vi "Prioritize LVCAM Error.vi"(10 "Error from LVCAM":errorcluster, 11 "Self Actor in":refnum<class "Self Actor.lvclass">) -> (3 "Self Actor out":refnum<class "Self Actor.lvclass">)   [LabVIEW 2021, in "LVCAM.lvlib" / "Self Actor.lvclass"]
uses:
  Self Actor.lvclass
  Self Actor.lvclass/Self Actor.ctl
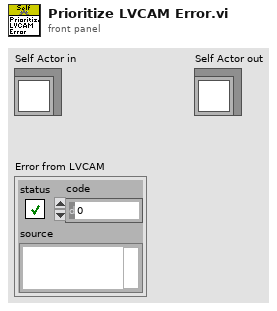
[diagram p1: front panel]
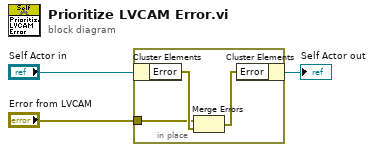
[diagram p0: block diagram]
diagram:
  n1 = in-place {
    in-place-border: "Error from LVCAM" -> [w4]
    n2 = in-place-cluster #1("Self Actor in") -> ("Error"=w6:errorcluster)
    n3 = Merge Errors(w4, w6) -> (w5:errorcluster)
    n4 = in-place-cluster #1("Error"=w5) -> (→"Self Actor out":refnum<class "Self Actor.lvclass">)
  }
